vi "CustCM-Save config.vi"(0 "configuration file path":path=path "C:/PXI Connections.txt", 1 "Pump Port":string, 5 "Analog Connections":cluster{"Outputs":string[], "Inputs":string[]}[](array[cluster]), 7 "Analog":cluster{"Inputs":string[], "Outputs":string[]}, 9 "Digital Connections":string[](array[string]), 11 "error in (no error)":errorcluster, 12 "Digital":cluster{"Inputs":string[], "Outputs":string[]}, 13 "Use 2090":bool, 14 "Hide unused":bool) -> (15 "error out":errorcluster)   [LabVIEW 2015]
uses:
  <vilib>/Utility/config.llb/Write Key (I32).vi
  <vilib>/Utility/config.llb/Write Key (Boolean).vi
  <vilib>/Utility/config.llb/Write Key (String).vi
  <vilib>/Utility/config.llb/NI_LVConfig.lvlib
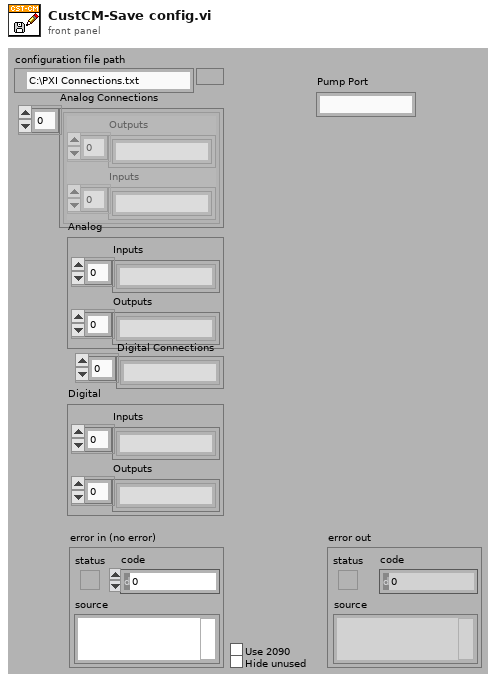
[diagram p1: front panel]
types:
  T1 = typedef "NI_LVConfig.lvlib/Config Data RefNum.ctl" = refnum<k1>
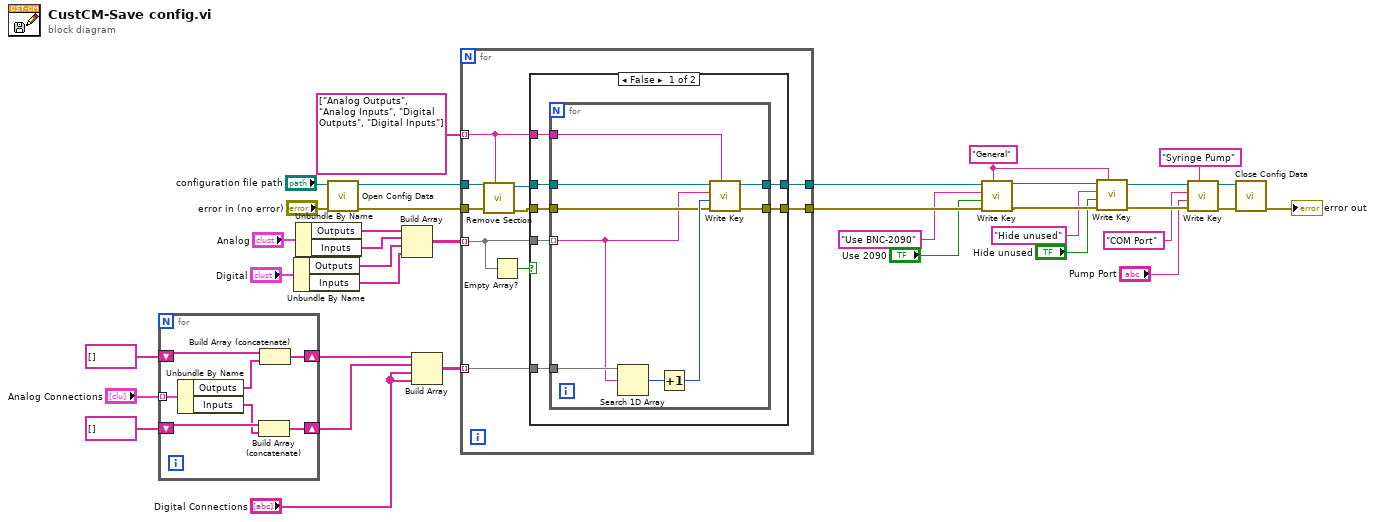
[diagram p0: block diagram]
diagram:
  w30 = "General" ("section")
  n1 = for {
    tunnel: "Analog Connections" -> [w43] mode=indexing
    shift-right: [w41] -> w14
    shift-left: string[] [] -> [w40]
    shift-right: [w39] -> w13
    shift-left: string[] [] -> [w38]
    n2 = Unbundle By Name(w43) -> ("Outputs"=w42:string[], "Inputs"=w37:string[])
    n3 = Build Array (concatenate)(w38, w37) -> (w39:string[])
    n4 = Build Array (concatenate)(w40, w42) -> (w41:string[])
  }
  n5 = Unbundle By Name("Digital") -> ("Outputs"=w10:string[], "Inputs"=w9:string[])
  n6 = Unbundle By Name("Analog") -> ("Outputs"=w20:string[], "Inputs"=w19:string[])
  n7 = call <vilib>:"Open Config Data.vi"("error in (no error)"="error in (no error)", "configuration file path"="configuration file path") -> ("error out"=w16:errorcluster, "refnum"=w17:T1)  [unwired: 7 in, 1 out]
  n8 = Build Array(w20, w19, w10, w9) -> (w15:string[][])
  n9 = Build Array(w14, w13, "Digital Connections", "Digital Connections") -> (w12:string[][])
  n10 = for {
    tunnel: [w53] -> w26
    tunnel: [w52] -> w25
    tunnel: string[] ["Analog Outputs", "Analog Inputs", "Digital Outputs", "Digital Inputs"] -> [w48] mode=indexing
    tunnel: w17 -> [w47]
    tunnel: w16 -> [w45]
    tunnel: w15 -> [w50] mode=indexing
    tunnel: w12 -> [w49] mode=indexing
    n11 = call <vilib>:"Remove Section.vi"("section"=w48, "error in (no error)"=w45, "refnum"=w47) -> ("error out"=w44:errorcluster, "refnum out"=w46:T1)  [unwired: 6 in, 1 out]
    n12 = Empty Array?(array=w50) -> (empty?=w51:bool)
    n13 = case shown="False" w51 {
      tunnel: w49 -> [w60 _]
      tunnel: w46 -> [w59 w71]
      tunnel: w44 -> [w58 w70]
      tunnel: w50 -> [w57 _]
      tunnel: [w56 w71] -> w53
      tunnel: [w55 w70] -> w52
      tunnel: w48 -> [w54 _]
      frame False {
        n14 = for {
          tunnel: w57 -> [w62] mode=indexing
          tunnel: w60 -> [w68]
          tunnel: w59 -> [w67]
          tunnel: [w64] -> w56
          tunnel: w58 -> [w65]
          tunnel: [w63] -> w55
          tunnel: w54 -> [w61]
          n15 = Search 1D Array(1D array=w68, element=w62) -> (index of element=w69:i32)  [unwired: 1 in]
          n16 = Increment(x=w69) -> (x+1=w66:i32)
          n17 = call-poly <vilib>:"Write Key.vi"("section"=w61, "error in (no error)"=w65, "value"=w66, "key"=w62, "refnum"=w67) -> ("error out"=w63:errorcluster, "refnum out"=w64:T1)  [unwired: 4 in, 1 out]
        }
      }
      frame True {
      }
    }
  }
  n18 = call-poly <vilib>:"Write Key.vi"("section"=w30, "error in (no error)"=w25, "value"="Use 2090", "key"="Use BNC-2090", "refnum"=w26) -> ("error out"=w29:errorcluster, "refnum out"=w28:T1)  [unwired: 4 in, 1 out]
  n19 = call-poly <vilib>:"Write Key.vi"("section"=w30, "error in (no error)"=w29, "value"="Hide unused", "key"="Hide unused", "refnum"=w28) -> ("error out"=w7:errorcluster, "refnum out"=w4:T1)  [unwired: 4 in, 1 out]
  n20 = call-poly <vilib>:"Write Key.vi"("section"="Syringe Pump", "error in (no error)"=w7, "value"="Pump Port", "key"="COM Port", "refnum"=w4) -> ("error out"=w6:errorcluster, "refnum out"=w5:T1)  [unwired: 4 in, 1 out]
  n21 = call <vilib>:"Close Config Data.vi"("error in (no error)"=w6, "refnum"=w5) -> ("error out"=→"error out":errorcluster)  [unwired: 8 in, 1 out]
